vi "get_corners.vi"(6 "error in (no error)":errorcluster, 9 "Station_Keeping in":refnum<class "Station_Keeping.lvclass">) -> (0 "error out":errorcluster, 1 "Buoy SE":cluster{"X":dbl, "Y":dbl}, 2 "Buoy NE":cluster{"X":dbl, "Y":dbl}, 3 "Station_Keeping out":refnum<class "Station_Keeping.lvclass">, 4 "Buoy SW":cluster{"X":dbl, "Y":dbl}, 5 "Buoy NW":cluster{"X":dbl, "Y":dbl})   [LabVIEW 2011, in "Station_Keeping.lvclass"]
uses:
  Station_Keeping.lvclass
  Station_Keeping.lvclass/Station_Keeping.ctl
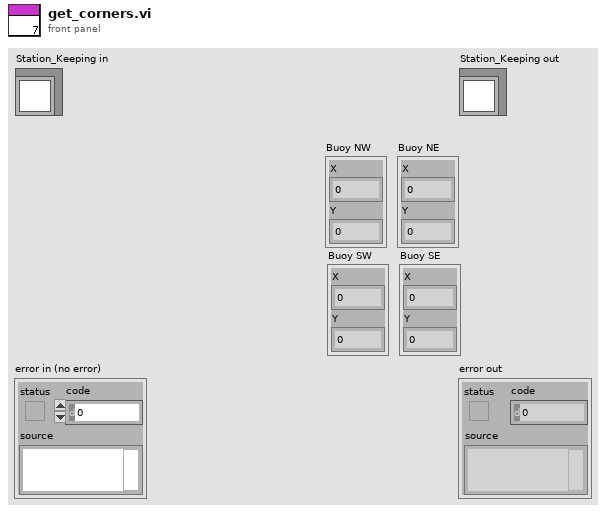
[diagram p1: front panel]
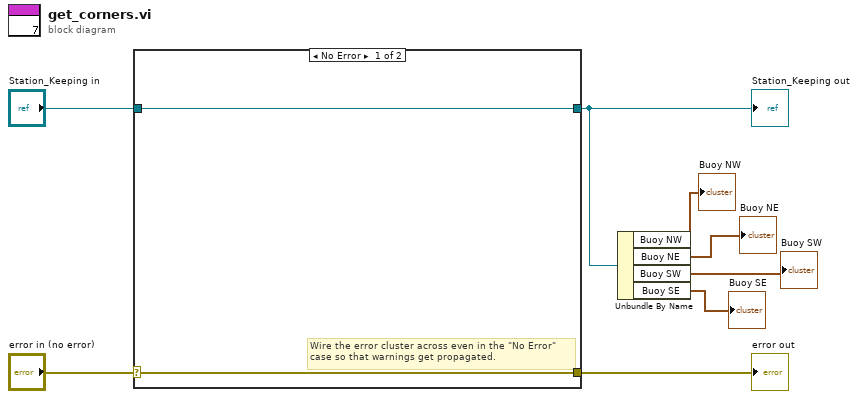
[diagram p0: block diagram]
diagram:
  n1 = case shown="No Error" "error in (no error)" {
    selector: "error in (no error)" -> [w9 w12]
    tunnel: [w9 w12] -> w7
    tunnel: [w10 w11] -> w5
    tunnel: "Station_Keeping in" -> [w10 w11]
    frame No Error {
      # "Wire the error cluster across even in the \"No Error\"\ncase so that warnings get propagated."
    }
    frame Error {
    }
  }
  "error out" <- w7
  "Station_Keeping out" <- w5
  n2 = Unbundle By Name(w5) -> ("Buoy NW"=→"Buoy NW":cluster{"X":dbl, "Y":dbl}, "Buoy NE"=→"Buoy NE":cluster{"X":dbl, "Y":dbl}, "Buoy SW"=→"Buoy SW":cluster{"X":dbl, "Y":dbl}, "Buoy SE"=→"Buoy SE":cluster{"X":dbl, "Y":dbl})
